vi "helloworld.vi"() -> ()   [LabVIEW 2017, in "gVision.lvlib"]
uses:
  gVision.lvlib
panel:
  out "return type":i32
  in  "x_fov":dbl=2000.0
  in  "error_bound":dbl=10.0
  in  "CDparam_1":i32=150
  in  "line_thickness":i32=2
  in  "CDred":i32
  in  "CDgreen":i32
  in  "CDblue":i32
  in  "circle_detection_sensitivity":i32=40
  in  "Picture size (between 0 and 1)":dbl=0.4
  in  "max_radius":i32=100
  in  "min_radius":i32=25
  in  "File Path":path=path "C:/Users/hayde/OneDrive/Desktop/Research Code/pick_and_place/fiducial_on_glass_74.png"
  # "7, 74 are good examples"
  # "For error circle"
  # "filepath for image"
  # "C:\\Users\\hayde\\OneDrive\\Desktop\\Research Code\\pick_and_place\\fiducial_on_glass_7.png"
  # "Circle Detection Parameters"
  # "in micrometers"
  # "warning, changing picture size affects circle detection!!"
  # "Max radius: 100 pixels is good"
  # "between 1 and 100,"
  # "small means it will detect everything, larger means stronger tolerance"
  # "all 0's for black"
  # "A gradient value that helps with edge detection"
  # "100 and 300 is a good range"
  # "between 1 and 5"
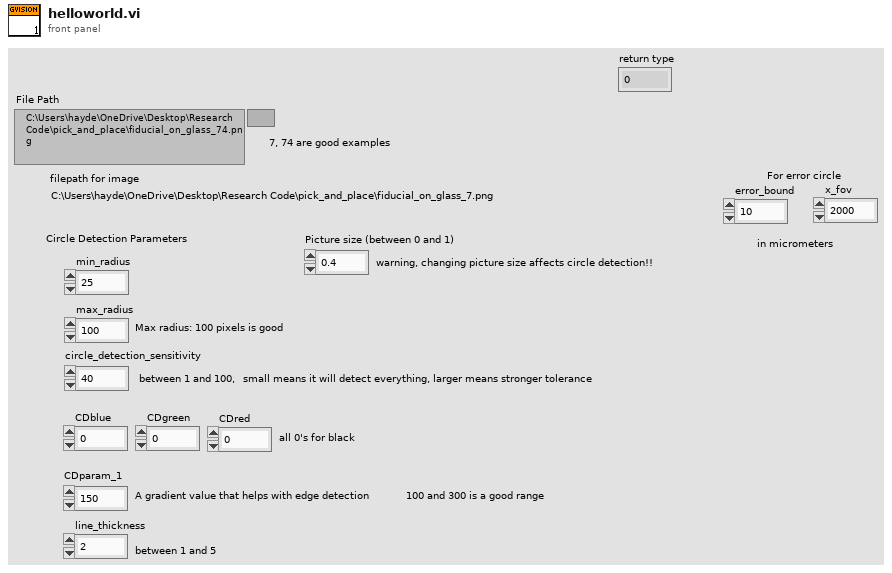
[diagram p1: front panel]
types:
  T1 = enum32{"Map Pixel Pointer", "Unmap Pixel Pointer", "Get Pixels Infos"}
  T2 = typedef "IMAQ Image.ctl" = refnum<image>
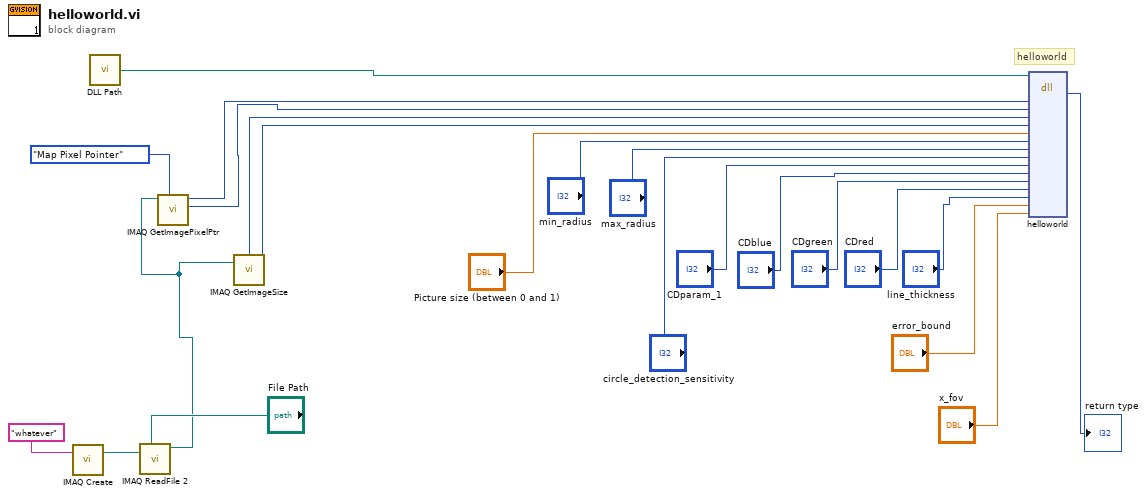
[diagram p0: block diagram]
diagram:
  # "helloworld"
  n1 = call "IMAQ Create"("Image Name"="whatever") -> ("New Image"=w21:T2)  [unwired: 4 in, 1 out]
  n2 = call "DLL Path.vi"() -> ("DLL Path"=w19:path)  [unwired: 5 in]
  n3 = call "IMAQ ReadFile 2"("File Path"="File Path", "Image"=w21) -> ("Image Out"=w11:T2)  [unwired: 5 in, 4 out]
  n4 = call "IMAQ GetImagePixelPtr"("Function"=T1."Map Pixel Pointer", "Image"=w11) -> ("LineWidth(Pixels)"=w12:i32, "Pixel Pointer out"=w17:u64)  [unwired: 4 in, 4 out]
  n5 = call "IMAQ GetImageSize"("Image"=w11) -> ("Y Resolution"=w15:i32, "X Resolution"=w16:i32)  [unwired: 3 in, 1 out]
  n6 = dll-call lib="?" fn="helloworld"(path in=w19, "img"=w17, "imgLineWidth"=w12, "imgWidth"=w16, "imgHeight"=w15, "percent_size"="Picture size (between 0 and 1)", "min_radius"="min_radius", "max_radius"="max_radius", "circle_detection_sensitivity"="circle_detection_sensitivity", "CDparam_1"="CDparam_1", "CDblue"="CDblue", "CDgreen"="CDgreen", "CDred"="CDred", "line_thickness"="line_thickness", "error_bound"="error_bound", "x_fov"="x_fov") -> ("return type"=→"return type":i32)  [unwired: 17 in, 2 out]
